vi "Anritsu VNA Set Sweep Time.vi"(6 "Channel":i8=1 min=1 step=1, 7 "Anritsu VNA":T1, 8 "error in (no error)":errorcluster, 10 "Sweep Time, s (-1: Auto)":dbl=-1.0, 11 "VISA Resource Name":refnum<visa-resource-name>) -> (0 "error out":errorcluster, 3 "dup VISA Resource Name":refnum<visa-resource-name>)   [LabVIEW 2011]
doc: "This Vi for the HP8753B Network Analyzer is used to set averaging, smoothing, and the IF bandwidth."
uses:
  TypeDefs/Anritsu VNA Instrument Info.ctl
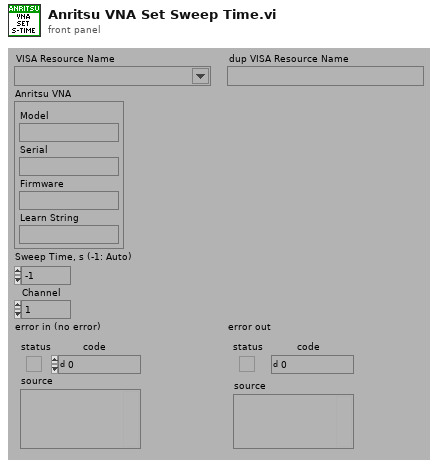
[diagram p1: front panel]
types:
  T1 = typedef "Anritsu VNA Instrument Info.ctl" = cluster{"Model":string, "Serial":string, "Firmware":string, "Learn String":string}
  T2 = typedef "Anritsu VNA Model.ctl" = enum16{"Not Supported", "37XXXX", "MS20XXX", "MS462XX", "MS464XX"}
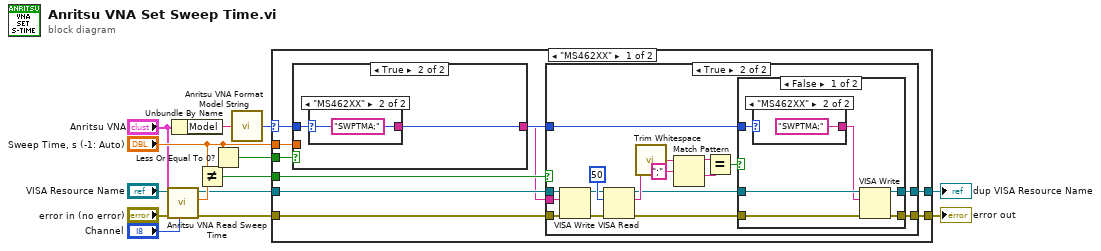
[diagram p0: block diagram]
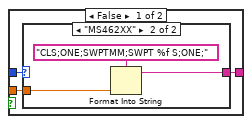
[diagram p5: hidden frame]
diagram:
  n1 = call "Anritsu VNA Read Sweep Time.vi"("Channel"="Channel", "Anritsu VNA"="Anritsu VNA", "error in (no error)"="error in (no error)", "VISA Resource Name"="VISA Resource Name") -> ("error out"=w5:errorcluster, "Sweep Time, s"=w12:dbl, "dup VISA Resource Name"=w4:refnum<visa-resource-name>)  [unwired: 5 out]
  n2 = Unbundle By Name("Anritsu VNA") -> ("Model"=w3:string)
  n3 = Not Equal?(x="Sweep Time, s (-1: Auto)", y=w12) -> (x != y?=w6:bool)
  n4 = Less Or Equal To 0?(x="Sweep Time, s (-1: Auto)") -> (x <= 0?=w7:bool)
  n5 = call "Anritsu VNA Format Model String.vi"("Model"=w3) -> ("Model"=w2:T2)
  n6 = case shown="\"MS462XX\"" w2 {
    selector: w2 -> [w20 _]
    tunnel: "Sweep Time, s (-1: Auto)" -> [w23 _]
    tunnel: w4 -> [w17 w61]
    tunnel: w5 -> [w15 w62]
    tunnel: [w21 w62] -> w9
    tunnel: [w22 w61] -> w8
    tunnel: w7 -> [w19 _]
    tunnel: w6 -> [w18 _]
    frame "MS462XX" {
      n7 = case shown="True" w19 {
        tunnel: w20 -> [w53 w59]
        tunnel: [w52 w58] -> w16
        tunnel: w23 -> [w54 _]
        frame False {
          n8 = case shown="\"MS462XX\"" w53 {
            tunnel: [_ w56] -> w52
            tunnel: w54 -> [_ w55]
            frame "Not Supported".."MS20XXX", "MS464XX" {
            }
            frame "MS462XX" {
              n9 = Format Into String(format string="CLS;ONE;SWPTMM;SWPT %f S;ONE;", w55) -> (resulting string=w56:string)  [unwired: 2 in, 1 out]
            }
          }
        }
        frame True {
          n10 = case shown="\"MS462XX\"" w59 {
            tunnel: [_ "SWPTMA;"] -> w58
            frame "Not Supported".."MS20XXX", "MS464XX" {
            }
            frame "MS462XX" {
            }
          }
        }
      }
      n11 = case shown="True" w18 {
        tunnel: w15 -> [w24 w29]
        tunnel: w17 -> [w25 w30]
        tunnel: [w25 w33] -> w22
        tunnel: [w24 w32] -> w21
        tunnel: w20 -> [_ w31]
        tunnel: w16 -> [_ w28]
        frame False {
        }
        frame True {
          n12 = VISA Write(VISA resource name=w30, write buffer=w28, error in (no error)=w29) -> (VISA resource name out=w27:refnum<visa-resource-name>, error out=w26:errorcluster)  [unwired: 1 out]
          n13 = VISA Read(VISA resource name=w27, byte count=u32 50, error in (no error)=w26) -> (VISA resource name out=w35:refnum<visa-resource-name>, read buffer=w40:string, error out=w34:errorcluster)  [unwired: 1 out]
          n14 = call <vilib>:"Trim Whitespace.vi"("string"=w40) -> ("trimmed string"=w39:string)  [unwired: 1 in]
          n15 = Match Pattern(string=w39, regular expression=";") -> (before substring=w38:string, after substring=w37:string)  [unwired: 3 out]
          n16 = Equal?(x=w38, y=w37) -> (x = y?=w36:bool)
          n17 = case shown="False" w36 {
            tunnel: w35 -> [w48 w51]
            tunnel: w34 -> [w47 w50]
            tunnel: [w46 w51] -> w33
            tunnel: [w45 w50] -> w32
            tunnel: w31 -> [w44 _]
            frame False {
              n18 = case shown="\"MS462XX\"" w44 {
                tunnel: [_ "SWPTMA;"] -> w43
                frame "Not Supported".."MS20XXX", "MS464XX" {
                }
                frame "MS462XX" {
                }
              }
              n19 = VISA Write(VISA resource name=w48, write buffer=w43, error in (no error)=w47) -> (VISA resource name out=w46:refnum<visa-resource-name>, error out=w45:errorcluster)  [unwired: 1 out]
            }
            frame True {
            }
          }
        }
      }
    }
    frame "Not Supported".."MS20XXX", "MS464XX" {
      # "These VNAs do not have the ability to set the sweep time."
    }
  }
  "error out" <- w9
  "dup VISA Resource Name" <- w8
